vi "Find Most Recent File.vi"(6 "pattern":string, 8 "error in (no error)":errorcluster, 11 "Folder Path":path) -> (0 "error out":errorcluster, 2 "Newest Path":path, 3 "dup Folder Path":path)   [LabVIEW 2019, in "Git.lvclass"]
uses:
  Git.lvclass
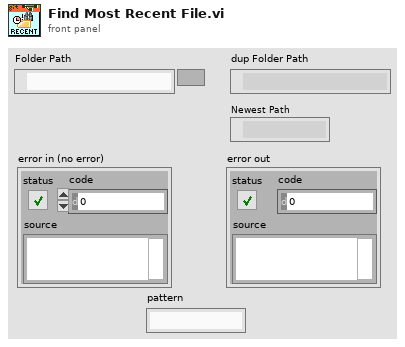
[diagram p1: front panel]
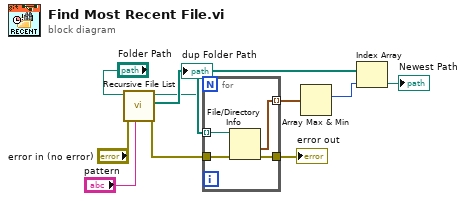
[diagram p0: block diagram]
diagram:
  n1 = call <vilib>:"Recursive File List.vi"("pattern"="pattern", "error in (no error)"="error in (no error)", "Folder Path"="Folder Path") -> ("error out"=w4:errorcluster, "All Files in Dir"=w3:path[], "dup Folder Path"=→"dup Folder Path":path)  [unwired: 4 in, 2 out]
  n2 = for {
    tunnel: w3 -> [w14] mode=indexing
    tunnel: [w13] -> w7 mode=indexing
    tunnel: w4 -> [w12]
    tunnel: [w11] -> w10
    n3 = File/Directory Info(path=w14, error in=w12) -> (last mod=w13:timestamp, error out=w11:errorcluster)  [unwired: 5 out]
  }
  "error out" <- w10
  n4 = Array Max & Min(array=w7) -> (max index (indices)=w8:i32)  [unwired: 3 out]
  n5 = Index Array(array=w3, index=w8) -> (element=→"Newest Path":path)
